vi "ConfigureDcMotorType.vi"(4 "error in (no error)":errorcluster, 6 "DC motor parameter":T1, 7 "axis in":cluster{"keyHandle":u32, "nodeId":u16}={"keyHandle"=0, "nodeId"=1}) -> (0 "error out":errorcluster, 3 "axis out":cluster{"keyHandle":u32, "nodeId":u16}={"keyHandle"=0, "nodeId"=1})   [LabVIEW 2019, in "maxonEPOS.lvlib"]
doc: "<B>ConfigureDcMotorType</B> writes the value for DC motor type to the device. Parameters for the DC motor type can be set."
uses:
  Examples/maxonEPOS.lvlib
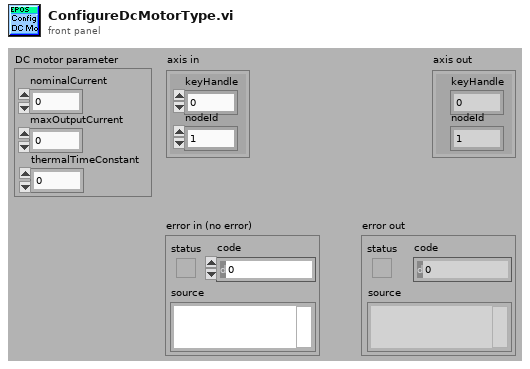
[diagram p1: front panel]
types:
  T1 = cluster{"nominalCurrent":u16, "maxOutputCurrent":u16, "thermalTimeConstant":u16}
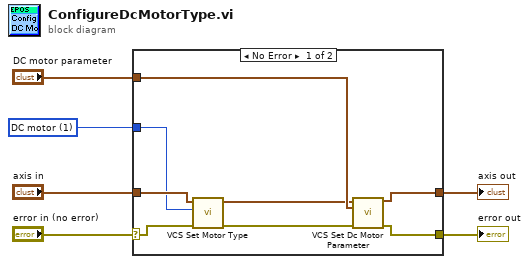
[diagram p0: block diagram]
diagram:
  w1 = u16 1 items=["DC motor"=1, "EC motor (sinus commutated)"=10, "EC motor (block commutated)"=11] ("motor type")
  n1 = case shown="No Error" "error in (no error)" {
    selector: "error in (no error)" -> [w14 w16]
    tunnel: [w13 w16] -> w5
    tunnel: [w12 w15] -> w4
    tunnel: "axis in" -> [w11 w15]
    tunnel: "DC motor parameter" -> [w10 _]
    tunnel: w1 -> [w9 _]
    frame No Error {
      n2 = call "VCS Set Motor Type.vi"("error in (no error)"=w14, "motor type"=w9, "axis in"=w11) -> ("error out"=w7:errorcluster, "axis out"=w8:cluster{"keyHandle":u32, "nodeId":u16})  [unwired: 7 in]
      n3 = call "VCS Set Dc Motor Parameter.vi"("axis in"=w8, "DC motor parameter"=w10, "error in (no error)"=w7) -> ("axis out"=w12:cluster{"keyHandle":u32, "nodeId":u16}, "error out"=w13:errorcluster)  [unwired: 11 in]
    }
    frame Error {
    }
  }
  "error out" <- w5
  "axis out" <- w4
